vi "stop.vi"(8 "error in (no error)":errorcluster, 11 "dummyCam in":refnum<class "dummyCam.lvclass">) -> (0 "error out":errorcluster, 3 "dummyCam out":refnum<class "dummyCam.lvclass">)   [LabVIEW 2018, in "dummyCam.lvclass"]
uses:
  dummyCam.lvclass
  globals/dummyTriggerVIref.vi
  _cameraBase/_cameraBase.lvclass
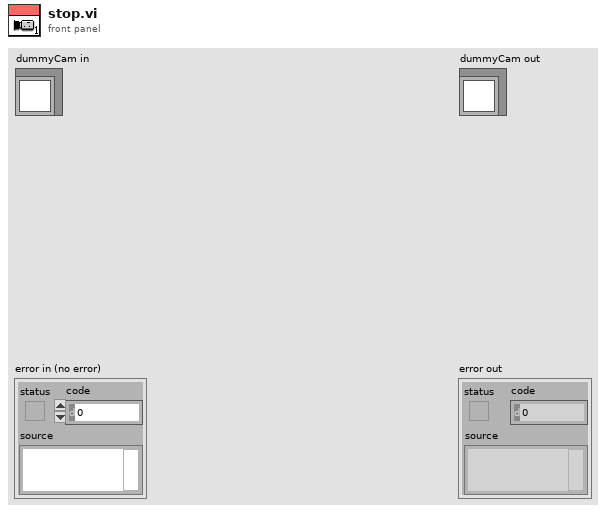
[diagram p1: front panel]
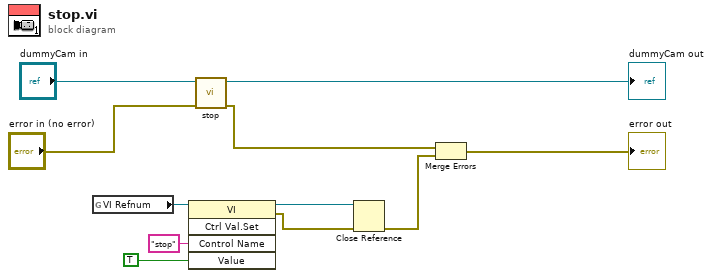
[diagram p0: block diagram]
diagram:
  n1 = global read "dummyTriggerVIref.vi" "VI Refnum"() -> (w8:refnum<vi>)
  n2 = invoke class="VI" method="Ctrl Val.Set"(reference=w8, "Control Name"="stop", "Value"=TRUE) -> (reference out=w5:refnum<vi>, error out=w4:errorcluster)  [unwired: 2 in, 3 out]
  n3 = call-parent "stop.vi"("error in (no error)"="error in (no error)", "_cameraBase in"="dummyCam in") -> ("error out"=w2:errorcluster, "_cameraBase out"=→"dummyCam out":refnum<class "dummyCam.lvclass">)  [unwired: 8 in]
  n4 = Close Reference(reference=w5, error in (no error)=w4) -> (error out=w3:errorcluster)
  n5 = Merge Errors(w2, w3) -> (→"error out":errorcluster)
